vi "Send Msg - Test.vi"() -> ()   [LabVIEW 2021]
uses:
  <vilib>/NI/STM/SubVIs/MetaDataElement.ctl
  <vilib>/NI/STM/TCP/Read Meta Data (TCP Ref).vi
  <vilib>/NI/STM/TCP/Get Connection Reference (TCP).vi
  <vilib>/NI/STM/TCP/Read Meta Data (TCP Clst).vi
  <vilib>/NI/STM/TCP/Write Message (TCP).vi
  <vilib>/NI/STM/NI STM.lvlib
  processes/ManageConnection/AudioGenManageConnection.lvlib
panel:
  out "connected":bool
  in  "stop":bool
  out "error out":errorcluster
  out "meta data":T1[](array[typedef])
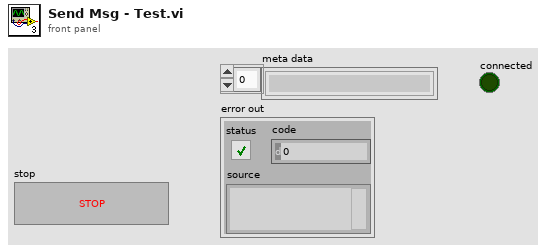
[diagram p1: front panel]
types:
  T1 = typedef "NI STM.lvlib/MetaDataElement.ctl" = string
  T2 = typedef "NI STM.lvlib/TCP Connection Info.ctl" = cluster{"connection ID":refnum<k5>, "meta data":T1[]}
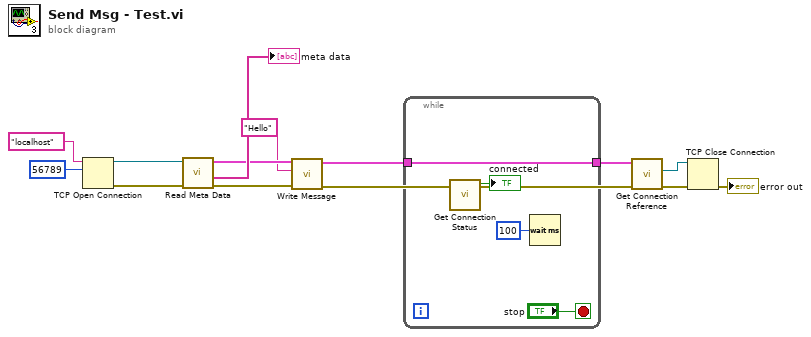
[diagram p0: block diagram]
diagram:
  n1 = TCP Open Connection(address="localhost" ("Target IP Address"), remote port or service name=u16 56789 ("remote port")) -> (connection ID=w14:refnum<k5>, error out=w13:errorcluster)  [unwired: 1 in, 2 out]
  n2 = call-poly <vilib>:"Read Meta Data.vi"("error in"=w13, "connection ID"=w14) -> ("error out"=w8:errorcluster, "meta data"=→"meta data":T1[], "connection info out"=w9:T2)  [unwired: 1 in, 6 out]
  n3 = call-poly <vilib>:"Write Message.vi"("error in"=w8, "name"="Hello", "connection info in"=w9) -> ("error out"=w4:errorcluster, "connection info out"=w2:T2)  [unwired: 2 in, 5 out]
  n4 = while {
    tunnel: w2 -> [w18]
    tunnel: [w18] -> w1
    stop <- "stop" stop-if-true
    n5 = call "Get Connection Status.vi"() -> ("connected"=→"connected":bool)  [unwired: 10 in, 1 out]
    n6 = Wait (ms)(milliseconds to wait=u32 100) -> ()  [unwired: 1 out]
  }
  n7 = call-poly <vilib>:"Get Connection Reference.vi"("error in"=w4, "connection info in"=w1) -> ("error out"=w5:errorcluster, "connection ID out"=w6:refnum<k5>)  [unwired: 8 out]
  n8 = TCP Close Connection(connection ID=w6, error in (no error)=w5) -> (error out=→"error out":errorcluster)  [unwired: 2 out]
